vi "MoveToEndStopSubVI.vi"(2 "error in (no error)":errorcluster, 3 "Boolean 2":refnum<vi>, 4 "LINX Resource":T1) -> (0 "error out":errorcluster, 1 "LINX Resource 2":T1)   [LabVIEW 2021]
uses:
  <vilib>/MakerHub/LINX/Private/Type Defs/LINX Ref.ctl
  <vilib>/MakerHub/LINX/Private/Type Defs/Platform.ctl
  <vilib>/MakerHub/LINX/Private/Type Defs/Interface.ctl
  <vilib>/MakerHub/LINX/Private/Device/Type Defs/LINX Device Config.ctl
  <vilib>/MakerHub/LINX/Private/Device/Type Defs/TCP Config.ctl
  <vilib>/MakerHub/LINX/Private/Device/Type Defs/Channels.ctl
  <vilib>/MakerHub/LINX/Public/Peripherals/Digital/Digital Write 1 Chan.vi
  <vilib>/MakerHub/LINX/Public/Peripherals/Digital/Digital Write N Chans.vi
  <vilib>/MakerHub/LINX/Private/Local IO/LinxDigitalWrite.vi
  <vilib>/MakerHub/LINX/Public/Utilities/Check Channel.vi
  <vilib>/MakerHub/LINX/Private/Utilties/Generate Error.vi
  <vilib>/MakerHub/LINX/LMH-LINX.lvlib
  <vilib>/MakerHub/LINX/Private/Device/Device.lvlib
panel:
  out "M0":bool=TRUE
  out "M1":bool=TRUE
  out "End Stop":bool
  in  "stop":bool
  # "Function & M0 & M1\n ----------------------\nFull  Step:       0         0\n1/2   Step:       1         0\n1/8   Step:       0         1\n1/16 Step:       1         1"
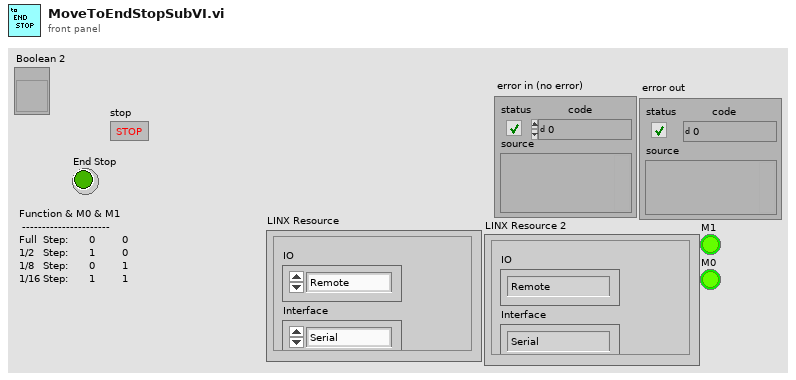
[diagram p1: front panel]
types:
  T1 = typedef "LMH-LINX.lvlib/LINX Ref.ctl" = cluster{"IO":T2, "Interface":T3, "LINX Device Config":T4}
  T2 = typedef "LMH-LINX.lvlib/Platform.ctl" = enum16{"Remote", "Local"}
  T3 = typedef "LMH-LINX.lvlib/Interface.ctl" = enum16{"Serial", "TCP"}
  T4 = typedef "LMH-LINX.lvlib/Device.lvlib/LINX Device Config.ctl" = cluster{"Interface":T3, "COM Port":refnum<visa-resource-name>, "TCP Configuration":T5, "Device Family":u8, "Device ID":u8, "Device Name":string, "TCP Ref":refnum<k5>, "Channels":T6}
  T5 = typedef "LMH-LINX.lvlib/Device.lvlib/TCP Config.ctl" = cluster{"IP Address":string, "Port":u16}
  T6 = typedef "LMH-LINX.lvlib/Channels.ctl" = cluster{"DI":u8[], "DO":u8[], "AI":u8[], "AO":u8[], "PWM":u8[], "QE":u8[], "UART":u8[], "I2C 2":u8[], "SPI":u8[], "CAN":u8[], "Servo":u8[], "AI Ref (V)":dbl, "AI Resolution (Bits)":u8, "AO Ref (V)":dbl, "AO Resolution (Bits)":u8}
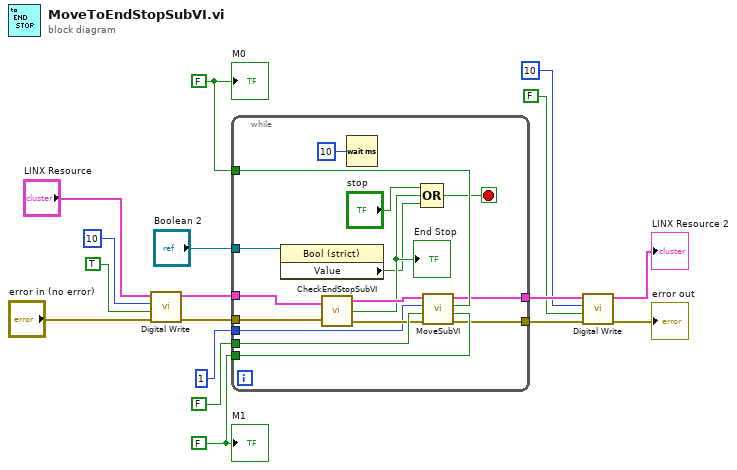
[diagram p0: block diagram]
diagram:
  w15 = FALSE ("M1")
  w16 = FALSE ("M0")
  n1 = call-poly <vilib>:"Digital Write.vi"("Error In"="error in (no error)", "Output Value"=TRUE, "DO Channel"=u8 10, "LINX Resource"="LINX Resource") -> ("Error Out"=w4:errorcluster, "LINX Resource"=w13:T1)  [unwired: 6 in]
  n2 = while {
    tunnel: FALSE ("Direction") -> [w33]
    tunnel: w16 -> [w32]
    tunnel: w15 -> [w31]
    tunnel: [w29] -> w12
    tunnel: [w27] -> w11
    tunnel: u32 1 ("Number of Steps") -> [w23]
    tunnel: w13 -> [w21]
    tunnel: w4 -> [w20]
    tunnel: "Boolean 2" -> [w19]
    stop <- w25 stop-if-true
    n3 = property class="Bool (strict)"(reference=w19) -> ("Value"=w18:bool)  [unwired: 1 in, 2 out]
    n4 = call "CheckEndStopSubVI.vi"("LINX Resource"=w21, "error in (no error)"=w20) -> ("LINX Resource 2"=w30:T1, "DI Value"=w24:bool, "error out"=w28:errorcluster)
    "End Stop" <- w24
    n5 = Wait (ms)(milliseconds to wait=u32 10) -> ()  [unwired: 1 out]
    n6 = Compound Arithmetic op=OR("stop", w24, w18) -> (w25:bool)
    n7 = call "MoveSubVI.vi"("M1"=w31, "M0"=w32, "error in (no error)"=w28, "Direction"=w33, "Number of Steps"=w23, "LINX Resource"=w30) -> ("error out"=w27:errorcluster, "LINX Resource 2"=w29:T1)
  }
  n8 = call-poly <vilib>:"Digital Write.vi"("Error In"=w11, "Output Value"=FALSE, "DO Channel"=u8 10, "LINX Resource"=w12) -> ("Error Out"=→"error out":errorcluster, "LINX Resource"=→"LINX Resource 2":T1)  [unwired: 6 in]
  "M1" <- w15
  "M0" <- w16
